vi "NT Get SubscribeHandle.vi"(4 "options":T1={"Send All"=FALSE, "Keep Duplicates"=FALSE, "rate (hz)"=10}, 8 "error in (no error)":errorcluster, 9 "description":string, 10 "NT_Type":T2 items=["NT_Unassigned"=0, "NT_Boolean"=1, "NT_Double"=2, "NT_String"=4, "NT_Raw"=8, "NT_BooleanArray"=16, "NT_DoubleArray"=32, "NT_StringArray"=64, "NT_RPC"=128, "NT_Integer"=256, "NT_Float"=512, "NT_IntegerArray"=1024, "NT_FloatArray"=2048], 11 "topicHandle":u32) -> (0 "error out":errorcluster, 3 "subscribeHandle":u32)   [LabVIEW 2025]
uses:
  <vilib>/Rock Robotics/Network Tables/NT Datatype.ctl
  <vilib>/Rock Robotics/Network Tables/NT SubscribeOptions.ctl
  FRC_NetworkTablesLV.dll
panel:
  in  "Remove":bool
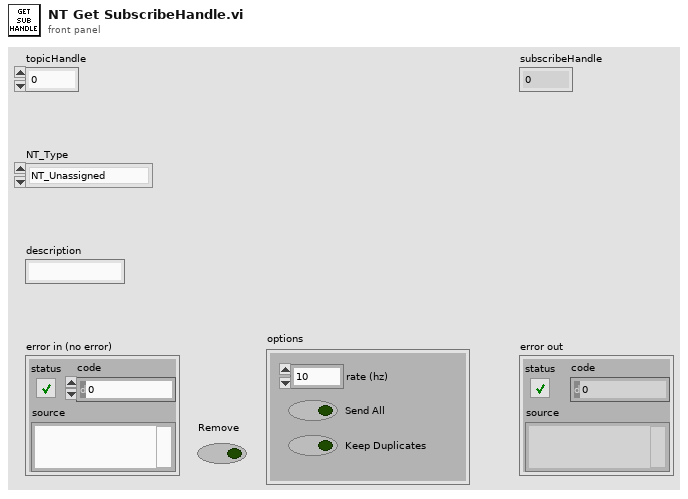
[diagram p1: front panel]
types:
  T1 = typedef "NT SubscribeOptions.ctl" = cluster{"Send All":bool, "Keep Duplicates":bool, "rate (hz)":u64}
  T2 = typedef "NT Datatype.ctl" = u32
  T3 = cluster{"size":u32, "poll":u32, "period":dbl, "exclude":u32, "sendAll":u32, "topicsOnly":u32, "prefixMatch":u32, "keepDups":u32, "disableRemote":u32, "disableLocal":u32, "excludeSelf":u32}
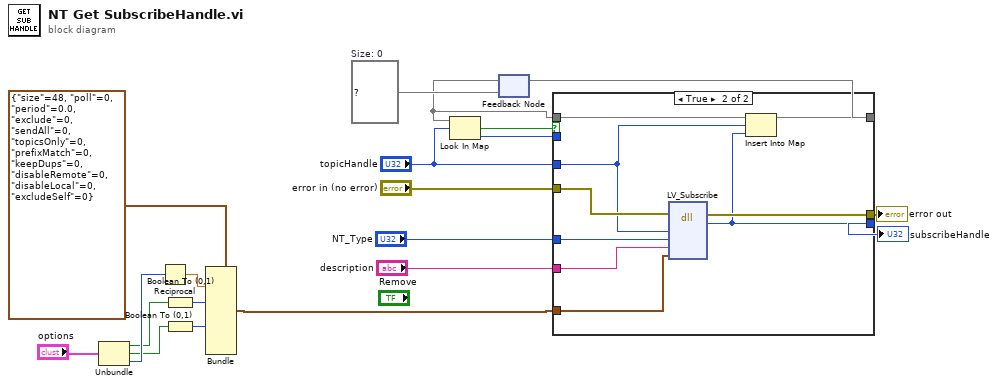
[diagram p0: block diagram]
diagram:
  w13 = map{u32, u32} {}  # Size: 0
  n1 = Unbundle("options") -> ("Send All"=w4:bool, "Keep Duplicates"=w2:bool, "rate (hz)"=w6:u64)
  n2 = Reciprocal(x=w6) -> (1/x=w7:dbl)
  n3 = Boolean To (0,1)(Boolean=w4) -> (0, 1=w5:i16)
  n4 = Boolean To (0,1)(Boolean=w2) -> (0, 1=w3:i16)
  n5 = Bundle(cluster=T3 {"size"=48, "poll"=0, "period"=0.0, "exclude"=0, "sendAll"=0, "topicsOnly"=0, "prefixMatch"=0, "keepDups"=0, "disableRemote"=0, "disableLocal"=0, "excludeSelf"=0}, "period"=w7, "sendAll"=w5, "keepDups"=w3) -> (w1:T3)  [unwired: 8 in]
  n6 = feedback #1(w13) -> (w11:map{u32, u32})
  n7 = Look In Map(map=w11, key="topicHandle") -> (key not found?=w14:bool, value=w12:u32)  [unwired: 1 in]
  n8 = case shown="True" w14 {
    tunnel: "description" -> [_ w32]
    tunnel: "topicHandle" -> [_ w26]
    tunnel: "error in (no error)" -> [w21 w31]
    tunnel: [w21 w30] -> w18
    tunnel: [w23 w25] -> w17
    tunnel: "NT_Type" -> [_ w29]
    tunnel: w12 -> [w23 _]
    tunnel: w11 -> [w22 w28]
    tunnel: [w22 w27] -> w10
    tunnel: w1 -> [_ w24]
    frame False {
    }
    frame True {
      n9 = dll-call lib="FRC_NetworkTablesLV.*" fn="LV_Subscribe"(error in=w31, "topicHandle"=w26, "type"=w29, "typeStr"=w32, "options"=w24) -> (error out=w30:errorcluster, "subscribeHandle"=w25:u32)  [unwired: 6 in, 1 out]
      n10 = Insert Into Map(map in=w28, key=w26, value=w25) -> (map out=w27:map{u32, u32})  [unwired: 2 out]
    }
  }
  "error out" <- w18
  "subscribeHandle" <- w17
  n11 = feedback-in #1(w10) -> ()
